vi "Register For Control Events.vi"(4 "Timeout [ms]":i32=-1, 6 "Timeout Message (to Self)":refnum<class "Message.lvclass">, 7 "Timeout Message Priority (Normal)":T1=enum."Normal", 8 "error in (no error)":errorcluster, 9 "Registration Types":T2[](array[typedef])=[enum."Value Change"], 10 "Control Refnums":refnum<vi>[](array[refnum]), 11 "IEventAggregator In":refnum<class "IEventAggregator.lvclass">) -> (0 "error out":errorcluster, 3 "IEventAggregator Out":refnum<class "IEventAggregator.lvclass">)   [LabVIEW 2015, in "ActorEvents.lvlib" / "IEventAggregator.lvclass"]
uses:
  IEventAggregator.lvclass
  <vilib>/event_ctls.llb/lveventtype.ctl
  <vilib>/ActorFramework/Message/Message.lvclass
  <vilib>/ActorFramework/Message Enqueuer/Message Priority.ctl
  IEventAggregator.lvclass/IEventAggregator.ctl
  IEventHandler/IEventHandler.lvclass/IEventHandler.ctl
  EventHandler/ControlEventHandler/ControlEventHandler.lvclass/ControlEventHandler.ctl
  IEventHandler/Write Registration Types.vi
  IEventHandler/Write Timeout Message.vi
  <vilib>/Utility/error.llb/Error Cluster From Error Code.vi
  EventHandler/ControlEventHandler/ControlEventHandler.lvclass
  IEventHandler/IEventHandler.lvclass
  <vilib>/ActorFramework/Message Enqueuer/Message Enqueuer.lvclass
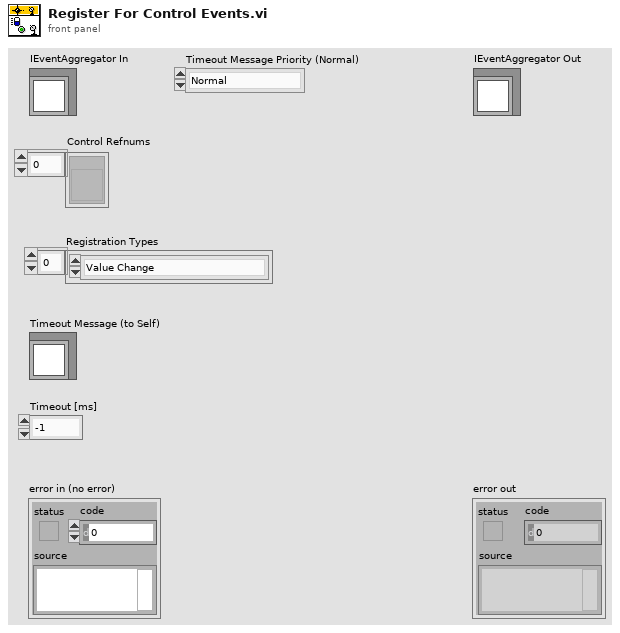
[diagram p1: front panel]
types:
  T1 = typedef "Actor Framework.lvlib/Message Enqueuer.lvclass/Message Priority.ctl" = enum16{"Low", "Normal", "High"}
  T2 = typedef "lveventtype.ctl" = enum32{"Null", "Timeout", "Annotation Menu Selection", "Annotation Menu Selection?", "App Instance Close", "App Instance Close?", "Autoscale Range Change", "Bookmark Info Change", "Cell Edit", "Cell Edit?", "Cursor Grab", "Cursor Grab?", "Cursor Menu Selection", "Cursor Menu Selection?", "Cursor Move", "Cursor Release", "Data Change", "Direction Change", "Display State Change", "Drag Ended", "Drag Enter", "Drag Leave", "Drag Over", "Drag Source Update", "Drag Starting", "Drag Starting?", "Drop", "Exec State Change", "Key Down", "Key Down?", "Key Repeat", "Key Repeat?", "Key Up", "Listbox Double Click", "Menu Activation?", "Menu Selection (App)", "Menu Selection? (App)", "Menu Selection (User)", "Mouse Down", "Mouse Down?", "Mouse Enter", "Mouse Leave", "Mouse Move", "Mouse Up", "Mouse Wheel", "NI Security User Change (App)", "Pane Size", "Panel Close", "Panel Close?", "Panel Resize", "Plot Attribute Change", "Scale Range Change", "Shortcut Menu Activation?", "Shortcut Menu Selection (App)", "Shortcut Menu Selection? (App)", "Shortcut Menu Selection (User)", "Tree Double Click", "Tree Drag", "Tree Drag?", "Tree Drop", "Tree Drop?", "Tree Item Close", "Tree Item Close?", "Tree Item Open", "Tree Item Open?", "User Event", "Value Change"}
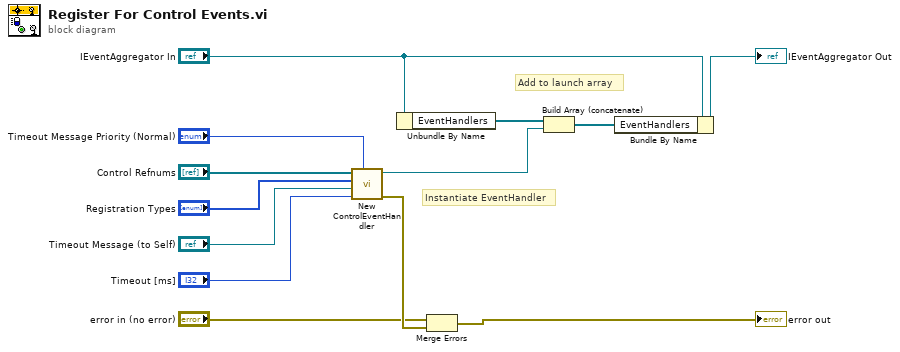
[diagram p0: block diagram]
diagram:
  # "Add to launch array"
  # "Instantiate EventHandler"
  n1 = call "New ControlEventHandler.vi"("Timeout Message Priority (Normal)"="Timeout Message Priority (Normal)", "Timeout [ms]"="Timeout [ms]", "Timeout Message"="Timeout Message (to Self)", "Registrations"="Registration Types", "Controls"="Control Refnums") -> ("error out"=w13:errorcluster, "ControlEventHandler"=w9:refnum<class "ControlEventHandler.lvclass">)  [unwired: 5 in]
  n2 = Unbundle By Name("IEventAggregator In") -> ("EventHandlers"=w11:refnum<class "IEventHandler.lvclass">[])
  n3 = Merge Errors("error in (no error)", w13) -> (→"error out":errorcluster)
  n4 = Build Array (concatenate)(w11, w9) -> (w10:refnum<class "IEventHandler.lvclass">[])
  n5 = Bundle By Name(cluster="IEventAggregator In", "EventHandlers"=w10) -> (→"IEventAggregator Out":refnum<class "IEventAggregator.lvclass">)
